vi "Insert Data.vi"(7 "Group":string, 8 "error in":errorcluster, 9 "Data":variant, 10 "tag":string, 11 "CVT Session In":T1) -> (0 "error out":errorcluster, 3 "CVT Session Out":T1)   [LabVIEW 2016, in "CVT.lvclass"]
uses:
  CVT.lvclass
  _Session Fwk/Typedefs/Session Handle.ctl
  _Session Fwk/Session - Root.lvclass
  G:/sw_repo/For Builds/Reusable/Session APIs/_Session Fwk/Session - Root.lvclass
  CVT.lvclass/CVT.ctl
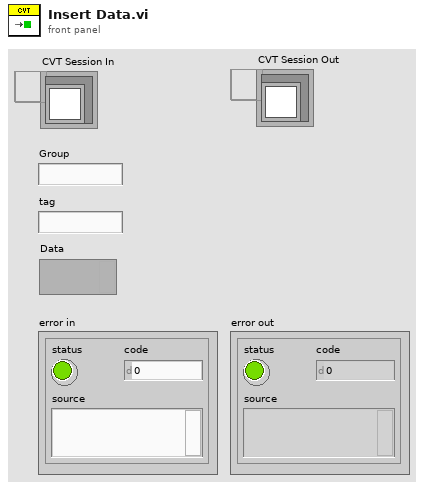
[diagram p1: front panel]
types:
  T1 = typedef "Session - Root.lvclass/Session Handle.ctl" = refnum<data-value>
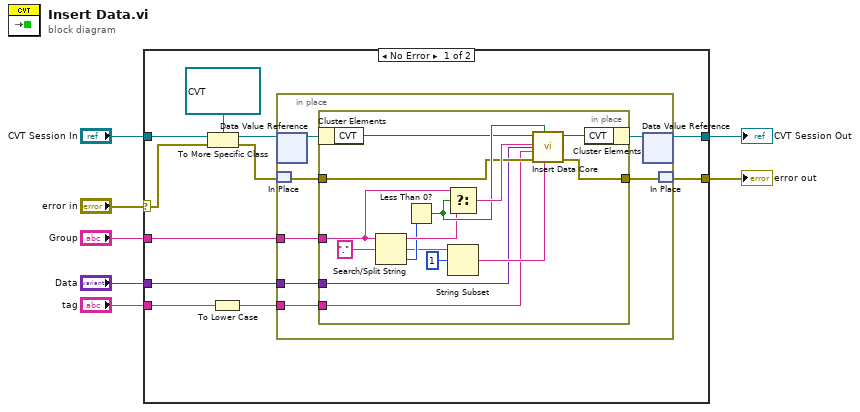
[diagram p0: block diagram]
diagram:
  n1 = case shown="No Error" "error in" {
    selector: "error in" -> [w8 w42]
    tunnel: "CVT Session In" -> [w18 w41]
    tunnel: "Data" -> [w15 _]
    tunnel: [w13 w41] -> w5
    tunnel: [w12 w42] -> w4
    tunnel: "Group" -> [w11 _]
    tunnel: "tag" -> [w10 _]
    frame No Error {
      n2 = To More Specific Class(target class=refnum<data-value> refnum ("CVT Session In"), reference=w18, error in=w8) -> (specific class reference=w16:refnum<data-value>, error out=w14:errorcluster)
      n3 = To Lower Case(string=w10) -> (all lower case string=w9:string)
      n4 = in-place {
        in-place-border: w11 -> [w25]
        in-place-border: w9 -> [w24]
        in-place-border: w15 -> [w23]
        n5 = in-place-dvr #1(w16) -> (w22:refnum<class "CVT.lvclass">)  [unwired: 1 out]
        n6 = in-place-match #2(w14) -> (w21:errorcluster)
        n7 = in-place {
          in-place-border: w25 -> [w27]
          in-place-border: w24 -> [w26]
          in-place-border: w23 -> [w28]
          in-place-border: w21 -> [w29]
          in-place-border: [w30] -> w19
          n8 = in-place-cluster #3(w22) -> ("CVT"=w32:variant)
          n9 = Search/Split String(string=w27, search string/char (-)="." ("regular expression")) -> (substring before match=w38:string, match + rest of string=w35:string, offset of match=w37:i32)  [unwired: 1 in]
          n10 = Less Than 0?(x=w37) -> (x < 0?=w39:bool)
          n11 = Select(t=w27, s=w39, f=w38) -> (s? t:f=w40:string)
          n12 = String Subset(string=w35, offset (0)=1) -> (substring=w33:string)  [unwired: 1 in]
          n13 = call "Insert Data Core.vi"("Data"=w28, "Nested Group"=w33, "Nested?"=w39, "error in"=w29, "tag"=w26, "Group"=w40, "CVT In"=w32) -> ("error out"=w30:errorcluster, "CVT Out"=w31:variant)  [unwired: 2 in]
          n14 = in-place-cluster #3("CVT"=w31) -> (w20:refnum<class "CVT.lvclass">)
        }
        n15 = in-place-dvr #1(w20) -> (w13:refnum<data-value>)  [unwired: 1 out]
        n16 = in-place-match #2(w19) -> (w12:errorcluster)
      }
    }
    frame Error {
      # "DO NOT UPDATE CVT IF ERROR WHEN TOGGLING VALUES"
    }
  }
  "CVT Session Out" <- w5
  "error out" <- w4
